vi "Allocate.vi"(8 "error in (no error)":errorcluster, 10 "size":u64 format="%d bytes", 11 "Pointer type":refnum<class "Pointer.lvclass">) -> (0 "error out":errorcluster, 3 "Pointer out":refnum<class "Pointer.lvclass">)   [LabVIEW 2020, in "Memory Manager.lvlib" / "Pointer.lvclass"]
doc: "Allocates a new pointer to a block of memory of <b>size</b> bytes."
uses:
  Pointer.lvclass
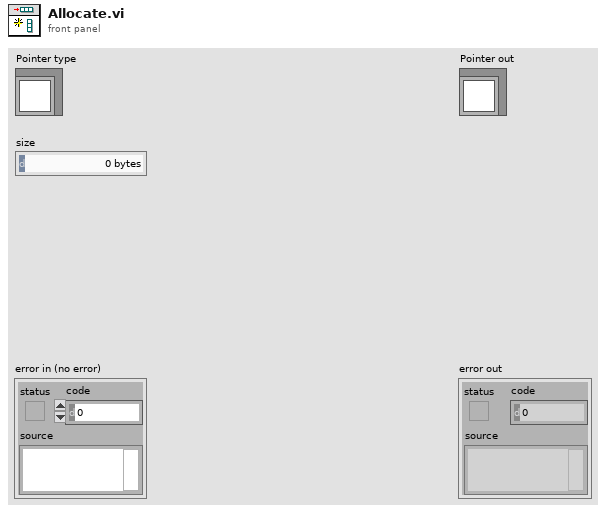
[diagram p1: front panel]
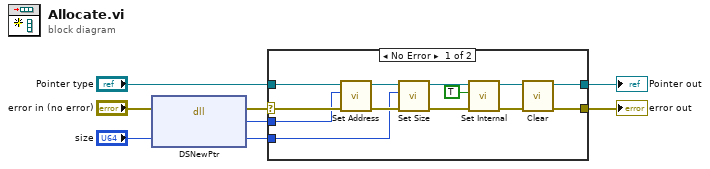
[diagram p0: block diagram]
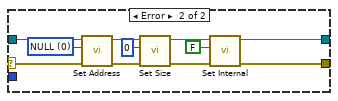
[diagram p2: hidden frame]
diagram:
  n1 = dll-call lib="LabVIEW" fn="DSNewPtr"(error in="error in (no error)", "size"="size") -> (error out=w6:errorcluster, "pointer"=w8:u64, "size"=w7:u64)  [unwired: 2 in, 1 out]
  n2 = case shown="No Error" w6 {
    selector: w6 -> [w12 w23]
    tunnel: "Pointer type" -> [w18 w24]
    tunnel: w8 -> [w10 _]
    tunnel: [w13 w20] -> w5
    tunnel: w7 -> [w9 _]
    tunnel: [w11 w23] -> w3
    frame No Error {
      n3 = call "Set Address.vi"("address"=w10, "Pointer in"=w18) -> ("Pointer out"=w17:refnum<class "Pointer.lvclass">)  [unwired: 9 in]
      n4 = call "Set Size.vi"("size"=w9, "Pointer in"=w17) -> ("Pointer out"=w16:refnum<class "Pointer.lvclass">)  [unwired: 9 in]
      n5 = call "Set Internal.vi"("internal"=TRUE, "Pointer in"=w16) -> ("Pointer out"=w14:refnum<class "Pointer.lvclass">)  [unwired: 9 in]
      n6 = call "Clear.vi"("error in (no error)"=w12, "Pointer in"=w14) -> ("error out"=w11:errorcluster, "Pointer out"=w13:refnum<class "Pointer.lvclass">)  [unwired: 8 in]
    }
    frame Error {
      w22 = u64 0 items=["NULL"] ("Null")
      n7 = call "Set Address.vi"("address"=w22, "Pointer in"=w24) -> ("Pointer out"=w25:refnum<class "Pointer.lvclass">)  [unwired: 9 in]
      n8 = call "Set Size.vi"("size"=u64 0, "Pointer in"=w25) -> ("Pointer out"=w21:refnum<class "Pointer.lvclass">)  [unwired: 9 in]
      n9 = call "Set Internal.vi"("internal"=FALSE, "Pointer in"=w21) -> ("Pointer out"=w20:refnum<class "Pointer.lvclass">)  [unwired: 9 in]
    }
  }
  "error out" <- w3
  "Pointer out" <- w5
